vi "SetOpenTime.vi"(8 "error in":errorcluster, 10 "OpenTime":timestamp, 11 "Defect in":refnum<class "Defect.lvclass">) -> (0 "error out":errorcluster, 3 "Defect out":refnum<class "Defect.lvclass">)   [LabVIEW 2021, in "ProligentXMLGenerator.lvlib" / "Defect.lvclass"]
doc: "Defines the creation time of the defect."
uses:
  Defect.lvclass
  Defect.lvclass/Defect.ctl
  Base/DateTime/DateTime.lvclass
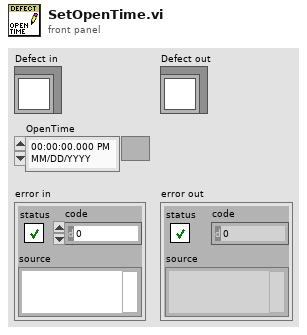
[diagram p1: front panel]
types:
  T1 = typedef "ProligentXMLGenerator.lvlib/Defect.lvclass/Data.ctl" = cluster{"Name":string, "Comments":refnum<class "UserComment.lvclass">[], "CustomData":refnum<class "CustomData.lvclass">, "DefectId":refnum<class "Guid.lvclass">, "OpenTime":refnum<class "DateTime.lvclass">, "TimeZoneInfoId":string}
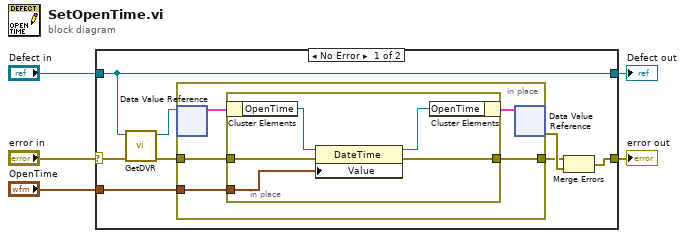
[diagram p0: block diagram]
diagram:
  n1 = case shown="No Error" "error in" {
    selector: "error in" -> [w11 w24]
    tunnel: "Defect in" -> [w6 w25]
    tunnel: [w8 w24] -> w3
    tunnel: "OpenTime" -> [w7 _]
    tunnel: [w6 w25] -> w1
    frame No Error {
      n2 = call "GetDVR.vi"("error in"=w11, "Defect"=w6) -> ("error out"=w10:errorcluster, "DVRReference"=w12:refnum<data-value>)  [unwired: 8 in]
      n3 = in-place "In Place Element Structure" {
        in-place-border: w10 -> [w18]
        in-place-border: [w17] -> w9
        in-place-border: w7 -> [w16]
        n4 = in-place-dvr #1(w12) -> (w15:T1)  [unwired: 1 out]
        n5 = in-place {
          in-place-border: w18 -> [w23]
          in-place-border: [w22] -> w17
          in-place-border: w16 -> [w19]
          n6 = in-place-cluster #2(w15) -> ("OpenTime"=w21:refnum<class "DateTime.lvclass">)
          n7 = property on="Property Node" class="DateTime"(reference=w21, error in=w23, "Value"=w19) -> (reference out=w20:refnum<class "DateTime.lvclass">, error out=w22:errorcluster)
          n8 = in-place-cluster #2("OpenTime"=w20) -> (w14:T1)
        }
        n9 = in-place-dvr #1(w14) -> (w13:errorcluster)  [unwired: 1 out]
      }
      n10 = Merge Errors(w9, w13) -> (w8:errorcluster)
    }
    frame Error {
    }
  }
  "error out" <- w3
  "Defect out" <- w1
